vi "Afterpulsing calculation big.vi"(10 "Histogram with 128 ns bin":i64[](array[numeric]), 11 "Total counts":i64) -> (3 "Afterpulsing probability (%)":dbl)   [LabVIEW 2012]
uses:
  <vilib>/Analysis/6fits.llb/Curve Fitting Criteria.ctl
  <vilib>/Analysis/NI_AALPro.lvlib
panel:
  out "Waveform Graph":dbl[][](graph)
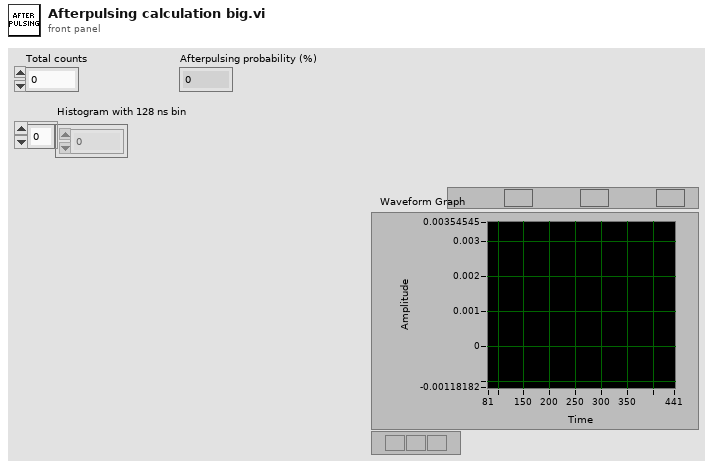
[diagram p1: front panel]
types:
  T1 = cluster{"amp min":dbl, "amp max":dbl, "damping min":dbl, "damping max":dbl, "offset min":dbl, "offset max":dbl}
  T2 = typedef "NI_AALPro.lvlib/Curve Fitting Criteria.ctl" = u16
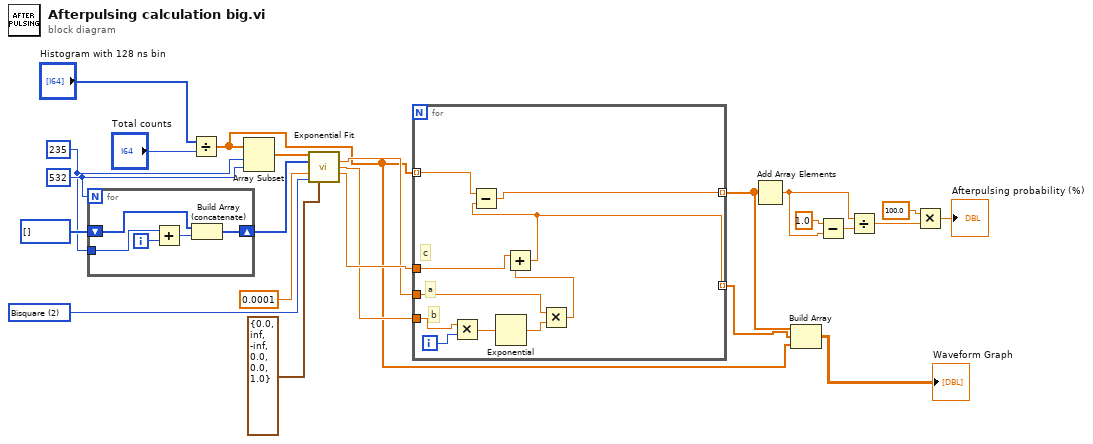
[diagram p0: block diagram]
diagram:
  w21 = T2 2 items=["Least Square", "Least Absolute Residual", "Bisquare"] ("method")
  w20 = 532 ("length")
  w9 = 235 ("index")
  n1 = for {
    N: w20 -> [_]
    shift-right: [w28] -> w13
    shift-left: i32[] [] -> [w26]
    tunnel: w9 -> [w24]
    i -> [w27]
    n2 = Add(x=w24, y=w27) -> (x+y=w25:i32)
    n3 = Build Array (concatenate)(w26, w25) -> (w28:i32[])
  }
  n4 = Divide(x="Histogram with 128 ns bin", y="Total counts") -> (x/y=w2:dbl[])
  n5 = Array Subset(array=w2, index=w9, length=w20) -> (w19:dbl[])
  n6 = call <vilib>:"Exponential Fit.vi"("Y"=w19, "X"=w13, "tolerance"=0.0001, "method"=w21, "parameter bounds"=T1 {"amp min"=0.0, "amp max"=inf, "damping min"=-inf, "damping max"=0.0, "offset min"=0.0, "offset max"=1.0}) -> ("amplitude"=w5:dbl, "damping"=w6:dbl, "offset"=w7:dbl)  [unwired: 5 in, 3 out]
  n7 = for {
    tunnel: w2 -> [w31] mode=indexing
    tunnel: w7 -> [w33]
    tunnel: w6 -> [w37]
    tunnel: w5 -> [w34]
    tunnel: [w30] -> w4 mode=indexing
    tunnel: [w29] -> w3 mode=indexing
    i -> [w38]
    # "b"
    # "a"
    # "c"
    n8 = Multiply(x=w37, y=w38) -> (x*y=w36:dbl)
    n9 = Exponential(1:w36) -> (0:w35:dbl)
    n10 = Multiply(x=w34, y=w35) -> (x*y=w32:dbl)
    n11 = Add(x=w33, y=w32) -> (x+y=w29:dbl)
    n12 = Subtract(x=w31, y=w29) -> (x-y=w30:dbl)
  }
  n13 = Add Array Elements(numeric array=w4) -> (sum=w8:dbl)
  n14 = Build Array(w4, w3, w2) -> (→"Waveform Graph":dbl[][])
  n15 = Subtract(x=1.0, y=w8) -> (x-y=w15:dbl)
  n16 = Divide(x=w8, y=w15) -> (x/y=w16:dbl)
  n17 = Multiply(x=100.0, y=w16) -> (x*y=→"Afterpulsing probability (%)":dbl)
